vi "Drive_Test.vi"(0 "Rotate Front Left":bool, 1 "Rotate Front Right":bool, 2 "Rotate Back Left":bool, 3 "Rotate Back Right":bool, 4 "Set_Wheel_Encoder_Positions":bool, 5 "Test_Joy_X":dbl, 6 "Test_Joy_Y":dbl, 8 "Zero_Gyro":bool) -> ()   [LabVIEW 2018]
uses:
  Subsytems/Drive/Drive_Notifier.ctl
  Subsytems/Drive/Drive_Control_Type.ctl
  Global_Variables/Drive_Globals.vi
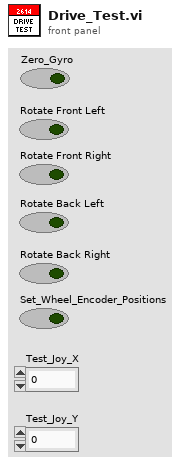
[diagram p1: front panel]
types:
  T1 = typedef "Drive_Notifier.ctl" = cluster{"Drive Control List":T2, "Front/Back":dbl, "Left/Right":dbl, "Turn":dbl, "Test_Joy_Y":dbl, "Test_Joy_X":dbl, "Set Wheel Encoder Positions":bool, "Robotcentric":bool, "Reset Gyro":bool, "Rotate Front Right":bool, "Rotate Front Left":bool, "Rotate Back Right":bool, "Rotate Back Left":bool}
  T2 = typedef "Drive_Control_Type.ctl" = enum16{"No_Op", "Set_Encoder_Positions", "Fieldcentric_PercentVBus", "Fieldcentric", "Robotcentric", "Reset_Gyro", "FR_Wheel", "FL_Wheel", "BR_Wheel", "BL_Wheel", "Manual_Wheel_Control"}
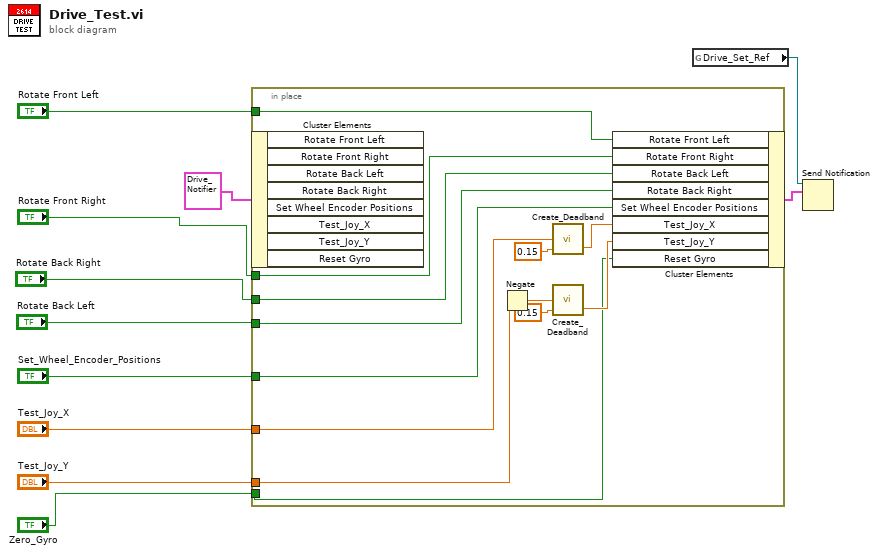
[diagram p0: block diagram]
diagram:
  n1 = in-place {
    in-place-border: "Rotate Front Left" -> [w20]
    in-place-border: "Rotate Front Right" -> [w19]
    in-place-border: "Rotate Back Right" -> [w18]
    in-place-border: "Rotate Back Left" -> [w17]
    in-place-border: "Set_Wheel_Encoder_Positions" -> [w16]
    in-place-border: "Test_Joy_X" -> [w15]
    in-place-border: "Test_Joy_Y" -> [w14]
    in-place-border: "Zero_Gyro" -> [w12]
    n2 = in-place-cluster #1 ("Unbundle / Bundle Elements")(T1 {"Drive Control List"=enum."No_Op", "Front/Back"=0.0, "Left/Right"=0.0, "Turn"=0.0, "Test_Joy_Y"=0.0, "Test_Joy_X"=0.0, "Set Wheel Encoder Positions"=FALSE, "Robotcentric"=FALSE, "Reset Gyro"=FALSE, "Rotate Front Right"=FALSE, "Rotate Front Left"=FALSE, "Rotate Back Right"=FALSE, "Rotate Back Left"=FALSE} ("Drive Notifier")) -> ()  [unwired: 8 out]
    n3 = Negate(x=w14) -> (-x=w13:dbl)
    n4 = call "Create_Deadband.vi"("Output Lower Limit"=0.15, "Input"=w15) -> ("Output"=w23:dbl)  [unwired: 1 in, 1 out]
    n5 = call "Create_Deadband.vi"("Output Lower Limit"=0.15, "Input"=w13) -> ("Output"=w21:dbl)  [unwired: 1 in, 1 out]
    n6 = in-place-cluster #1("Rotate Front Left"=w20, "Rotate Front Right"=w19, "Rotate Back Left"=w18, "Rotate Back Right"=w17, "Set Wheel Encoder Positions"=w16, "Test_Joy_X"=w23, "Test_Joy_Y"=w21, "Reset Gyro"=w12) -> (w11:T1)
  }
  n7 = global read "Drive_Globals.vi" "Drive_Set_Ref"() -> (w9:refnum<notifier>)
  n8 = Send Notification(notification=w11, notifier=w9) -> ()  [unwired: 1 in, 2 out]
